vi "Merge Rx Channels.vi"(9 "message":T1 {"Rx status handles" format="%.0x"; "Tx status handles" format="%.0x"; "timestamps" format="%.0x"; "parameters"."RxBC channel handle" format="%.0x"; "parameters"."RxRT channel handle" format="%.0x"; "parameters"."Tx channel handle" format="%.0x"}, 10 "RxBC channel handles":T3[](array[typedef]) format="%.0x", 11 "RxRT channel handles":T3[](array[typedef]) format="%.0x") -> (3 "Rx channel handles":T3[](array[typedef]) format="%.0x")   [LabVIEW 2020, in "AIM MIL-STD-1553 Engine.lvlib" / "Implementation.lvlib" / "Execution Unit.lvclass"]
uses:
  Execution Unit.lvclass
  <vilib>/NI VeriStand/Custom Device API/Custom Device Item Ref.ctl
  Message Handles.ctl
  Parameter Handles.ctl
  <vilib>/NI VeriStand/Custom Device API/Custom Device API.lvlib
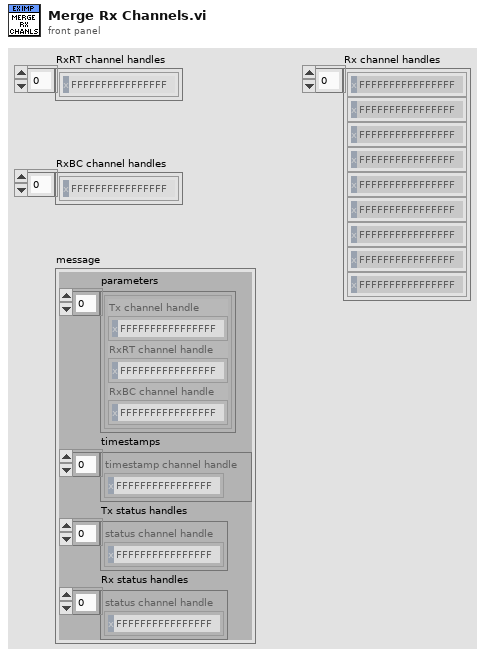
[diagram p1: front panel]
types:
  T1 = typedef "AIM MIL-STD-1553 Engine.lvlib/Implementation.lvlib/Execution Unit.lvclass/Message Handles.ctl" = cluster{"parameters":T2[], "timestamps":T3[], "Tx status handles":T3[], "Rx status handles":T3[]}
  T2 = typedef "AIM MIL-STD-1553 Engine.lvlib/Implementation.lvlib/Execution Unit.lvclass/Parameter Handles.ctl" = cluster{"Tx channel handle":T3, "RxRT channel handle":T3, "RxBC channel handle":T3}
  T3 = typedef "Custom Device API.lvlib/Custom Device Item Ref.ctl" = u64
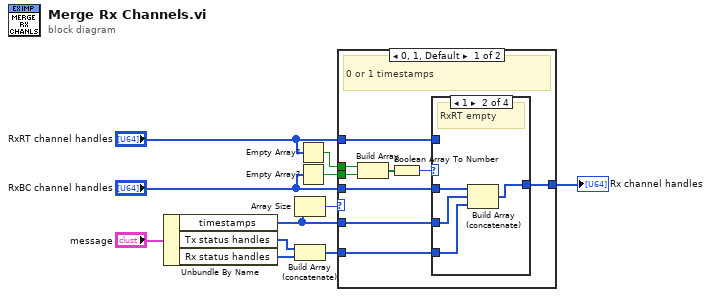
[diagram p0: block diagram]
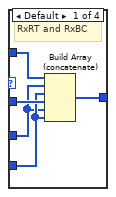
[diagram p2: hidden frame]
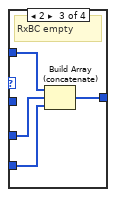
[diagram p3: hidden frame]
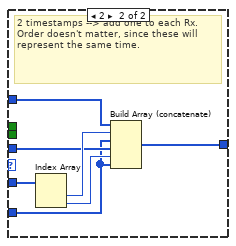
[diagram p5: hidden frame]
diagram:
  n1 = Unbundle By Name("message") -> ("timestamps"=w3:T3[], "Tx status handles"=w2:T3[], "Rx status handles"=w1:T3[])
  n2 = Array Size(array=w3) -> (size(s)=w11:i32)
  n3 = Build Array (concatenate)(w2, w1) -> (w9:T3[])
  n4 = Empty Array?(array="RxRT channel handles") -> (empty?=w7:bool)
  n5 = Empty Array?(array="RxBC channel handles") -> (empty?=w5:bool)
  n6 = case shown="0, 1, Default" w11 {
    tunnel: "RxRT channel handles" -> [w18 w40]
    tunnel: "RxBC channel handles" -> [w17 w38]
    tunnel: [w20 w36] -> w10
    tunnel: w3 -> [w16 w41]
    tunnel: w9 -> [w19 w35]
    tunnel: w5 -> [w14 _]
    tunnel: w7 -> [w15 _]
    frame 0, 1, Default {
      # "0 or 1 timestamps"
      n7 = Build Array(w15, w14) -> (w13:bool[])
      n8 = Boolean Array To Number(Boolean array=w13) -> (number=w12:u32)
      n9 = case shown="1" w12 {
        tunnel: w17 -> [w25 w29 _ _]
        tunnel: [w24 w28 w33 w34] -> w20
        tunnel: w19 -> [w23 w27 w32 w34]
        tunnel: w18 -> [w22 _ w31 _]
        tunnel: w16 -> [w21 w26 w30 _]
        frame Default {
          # "RxRT and RxBC"
          n10 = Build Array (concatenate)(w22, w21, w23, w25, w21, w23) -> (w24:T3[])
        }
        frame 1 {
          # "RxRT empty"
          n11 = Build Array (concatenate)(w29, w26, w27) -> (w28:T3[])
        }
        frame 2 {
          # "RxBC empty"
          n12 = Build Array (concatenate)(w31, w30, w32) -> (w33:T3[])
        }
        frame 3 {
          # "No Rx channels"
        }
      }
    }
    frame 2 {
      # "2 timestamps --> add one to each Rx. Order doesn't matter, since these will represent the same time."
      n13 = Index Array(array=w41) -> (element #1=w39:T3, element #2=w37:T3)  [unwired: 2 in]
      n14 = Build Array (concatenate)(w40, w39, w35, w38, w37, w35) -> (w36:T3[])
    }
  }
  "Rx channel handles" <- w10
